vi "Configure FFT Measurement Trigger Gap.vi"(8 "error in (no error)":errorcluster, 9 "Gap (0.0)":dbl format="%^.3e", 10 "Instance (1)":i32=1, 11 "VISA resource name":refnum<visa-resource-name>) -> (0 "error out":errorcluster, 3 "VISA resource name out":refnum<visa-resource-name>)   [LabVIEW 2020, in "Rohde&Schwarz CMXP GPRF.lvlib"]
doc: "Defines a minimum duration of the power-down periods (gaps) between two triggered IF power pulses.\n\nAttribute:\nRSCMXPGPRF_ATTR_FFT_MEASUREMENT_TRIGGER_GAP\n\nRemote-control command:\nTRIGger:GPRF:MEAS<i>:FFTSanalyzer:MGAP"
uses:
  <instrlib>/Rohde&Schwarz CMXP GPRF/Rohde&Schwarz CMXP GPRF.lvlib
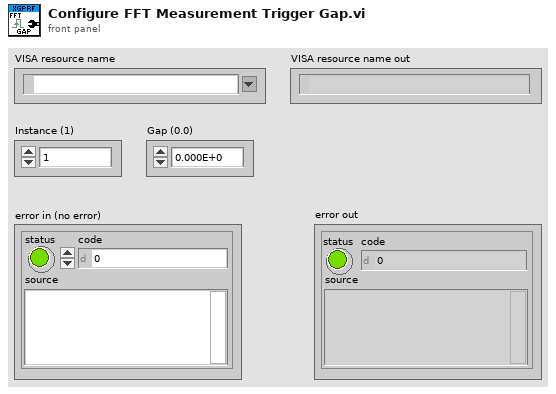
[diagram p1: front panel]
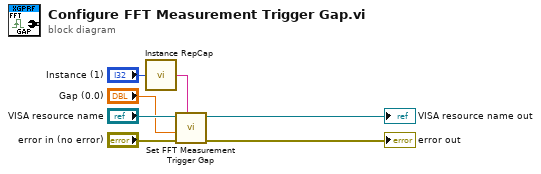
[diagram p0: block diagram]
diagram:
  n1 = call <instrlib>:"Instance RepCap.vi"("Instance in"="Instance (1)") -> ("Instance out"=w4:string)
  n2 = call "Set FFT Measurement Trigger Gap"("Repeated Capabilities"=w4, "error in (no error)"="error in (no error)", "FFT Measurement Trigger Gap (0.0)"="Gap (0.0)", "instrument handle"="VISA resource name") -> ("error out"=→"error out":errorcluster, "instrument handle out"=→"VISA resource name out":refnum<visa-resource-name>)  [unwired: 6 in]
